vi "DAC Init Results.vi"(8 "error in":errorcluster, 9 "Log Details?":bool, 10 "tdms file":refnum<k34>, 11 "DAC Traverse in":refnum<class "DAC Traverse.lvclass">) -> (0 "error out":errorcluster, 2 "tdms file out":refnum<k34>)   [LabVIEW 2019, in "DAC.lvlib" / "DAC Traverse.lvclass"]
uses:
  DAC Traverse.lvclass
  C:/Users/wg/Documents/LV_Projects/test-stand/App/DAC/DAC.lvclass
  DAC.lvclass/DAC.ctl
  DAC Traverse.lvclass/DAC Traverse.ctl
  DAC.lvclass
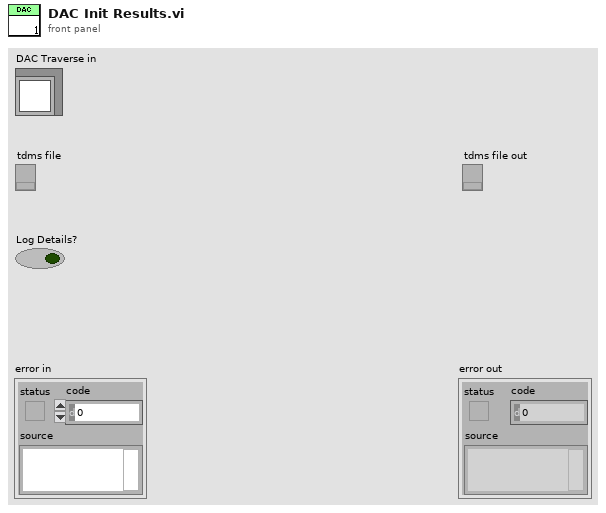
[diagram p1: front panel]
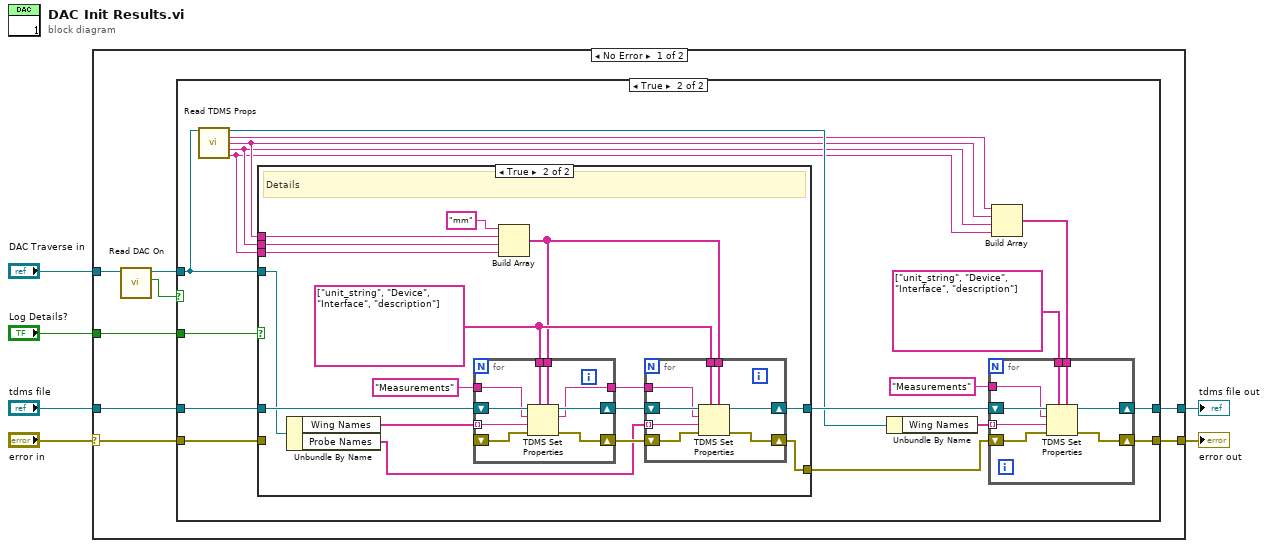
[diagram p0: block diagram]
diagram:
  n1 = case shown="No Error" "error in" {
    selector: "error in" -> [w8 w78]
    tunnel: [w12 w78] -> w3
    tunnel: "DAC Traverse in" -> [w11 _]
    tunnel: "tdms file" -> [w14 w77]
    tunnel: [w13 w77] -> w2
    tunnel: "Log Details?" -> [w7 _]
    frame No Error {
      n2 = call "Read DAC On.vi"("DAC in"=w11) -> ("DAC On"=w9:bool, "DAC out"=w10:refnum<class "DAC Traverse.lvclass">)  [unwired: 8 in, 1 out]
      n3 = case shown="True" w9 {
        tunnel: w14 -> [w16 w29]
        tunnel: [w16 w33] -> w13
        tunnel: [w15 w32] -> w12
        tunnel: w10 -> [_ w24]
        tunnel: w8 -> [w15 w25]
        tunnel: w7 -> [_ w30]
        frame False {
        }
        frame True {
          n4 = call "Read TDMS Props.vi"("DAC in"=w24) -> ("DAC out"=w23:refnum<class "DAC Traverse.lvclass">, "Result Unit"=w22:string, "DAC Device"=w21:string, "DAC IO"=w20:string, "DAC Description"=w19:string)  [unwired: 10 in]
          n5 = case shown="True" w30 {
            tunnel: w29 -> [w35 w51]
            tunnel: [w35 w45] -> w28
            tunnel: w24 -> [_ w50]
            tunnel: [w34 w47] -> w26
            tunnel: w25 -> [w34 _]
            tunnel: w21 -> [_ w38]
            tunnel: w20 -> [_ w37]
            tunnel: w19 -> [_ w36]
            frame False {
            }
            frame True {
              w40 = string[] ["unit_string", "Device", "Interface", "description"] ("property names")
              # "Details"
              n6 = Unbundle By Name(w50) -> ("Wing Names"=w42:string[], "Probe Names"=w41:string[])
              n7 = Build Array("mm" ("element"), w38, w37, w36) -> (w39:string[])
              n8 = for {
                tunnel: w40 -> [w67]
                tunnel: w39 -> [w66]
                shift-right: [w65] -> w46
                shift-left: w51 -> [w68]
                tunnel: "Measurements" ("group name in (Untitled)") -> [w63]
                shift-right: [w64] -> w48
                shift-left: _ -> [w62]
                tunnel: w42 -> [w61] mode=indexing
                tunnel: [w60] -> w44
                n9 = TDMS Set Properties(5:w66, 7:w67, 8:w62, 9:w61, 10:w63, 11:w68) -> (0:w64:errorcluster, 2:w60:string, 3:w65:refnum<k34>)  [unwired: 1 out]
              }
              n10 = for {
                tunnel: w40 -> [w58]
                tunnel: w39 -> [w57]
                shift-right: [w56] -> w45
                shift-left: w46 -> [w59]
                tunnel: w44 -> [w54]
                shift-right: [w55] -> w47
                shift-left: w48 -> [w53]
                tunnel: w41 -> [w52] mode=indexing
                n11 = TDMS Set Properties(5:w57, 7:w58, 8:w53, 9:w52, 10:w54, 11:w59) -> (0:w55:errorcluster, 3:w56:refnum<k34>)  [unwired: 2 out]
              }
            }
          }
          n12 = Unbundle By Name(w23) -> ("Wing Names"=w31:string[])
          n13 = Build Array(w22, w21, w20, w19) -> (w17:string[])
          n14 = for {
            tunnel: w31 -> [w75] mode=indexing
            tunnel: string[] ["unit_string", "Device", "Interface", "description"] ("property names") -> [w74]
            tunnel: w17 -> [w73]
            shift-right: [w72] -> w33
            shift-left: w28 -> [w76]
            tunnel: "Measurements" ("group name in (Untitled)") -> [w70]
            shift-right: [w71] -> w32
            shift-left: w26 -> [w69]
            n15 = TDMS Set Properties(5:w73, 7:w74, 8:w69, 9:w75, 10:w70, 11:w76) -> (0:w71:errorcluster, 3:w72:refnum<k34>)  [unwired: 2 out]
          }
        }
      }
    }
    frame Error {
    }
  }
  "error out" <- w3
  "tdms file out" <- w2
